vi "Global Var.vi"() -> ()   [LabVIEW 2014]
panel:
  in  "Auto_Cans Delay":bool
  in  "Wips_Auto":bool
  in  "Auto_Cans":bool
  in  "Auto_3_tote":bool
  in  "Auto_Select":bool
  in  "Store_High":bool
  in  "Can_Door":bool
  in  "Master_Auto_Stop":bool
  in  "Yoyo_Pos_Light":dbl
  in  "Light_Show":bool
  in  "Auto 15":bool
  in  "Auto 14":bool
  in  "Auto 13":bool
  in  "Auto 12":bool
  in  "Auto 11":bool
  in  "Auto 10":bool
  in  "Auto 9":bool
  in  "Auto 8":bool
  in  "Auto 7":bool
  in  "Auto 6":bool
  in  "Auto 5":bool
  in  "Auto 4":bool
  in  "Auto 3":bool
  in  "Auto 2":bool
  in  "Auto":bool
  in  "Encoder_Dist":dbl
  in  "Auto_Tote_Picked_Up":bool
  in  "Auto_Infeed_Ben":bool
  in  "Auto_Master_Stop_Value":bool
  in  "Auto_Drive_No_PID_Power":dbl
  in  "Auto_Turn_No_PID_Power":dbl
  in  "Auto_Drive_No_PID_Enable":bool
  in  "Auto_Drive_Straight_Power":dbl
  in  "Auto_Drive_Straight_Enable":bool
  in  "Auto_State":dbl
  in  "Floor_Tote_Detected":bool
  in  "Step_1":bool
  in  "Can_Tip_Flip":bool
  in  "Can_Tip_Arm":bool
  in  "Infeed_Open":bool
  in  "Step_3":bool
  in  "Carry":bool
  in  "Eject_Manual":dbl
  in  "Score_Step":bool
  in  "Score_Tote":dbl
  in  "Reset_Encoder":bool
  in  "Ele_Pos_Yoyo":dbl
  in  "Right_Dist":dbl
  in  "Left_Dist":dbl
  in  "Arm_Pos":bool
  in  "Step_Pos":bool
  in  "Eject_Out":dbl
  in  "Eject_In":dbl
  in  "Reset_Yaw":bool
  in  "Yaw":dbl
  in  "Store_Pos":bool
  in  "Exit_Pos":bool
  in  "Infeed":dbl
  in  "Elevator":dbl
  in  "Station_Pickup":bool
  in  "Floor_Pickup":bool
  in  "Turnin_Main":dbl
  in  "Turning_Limit":dbl
  in  "Speed_Main":dbl
  in  "Speed_Limit":dbl
  # "Auto"
  # "Automation"
  # "Drive Motors"
  # "Sensors"
  # "Positions"
  # "Imp"
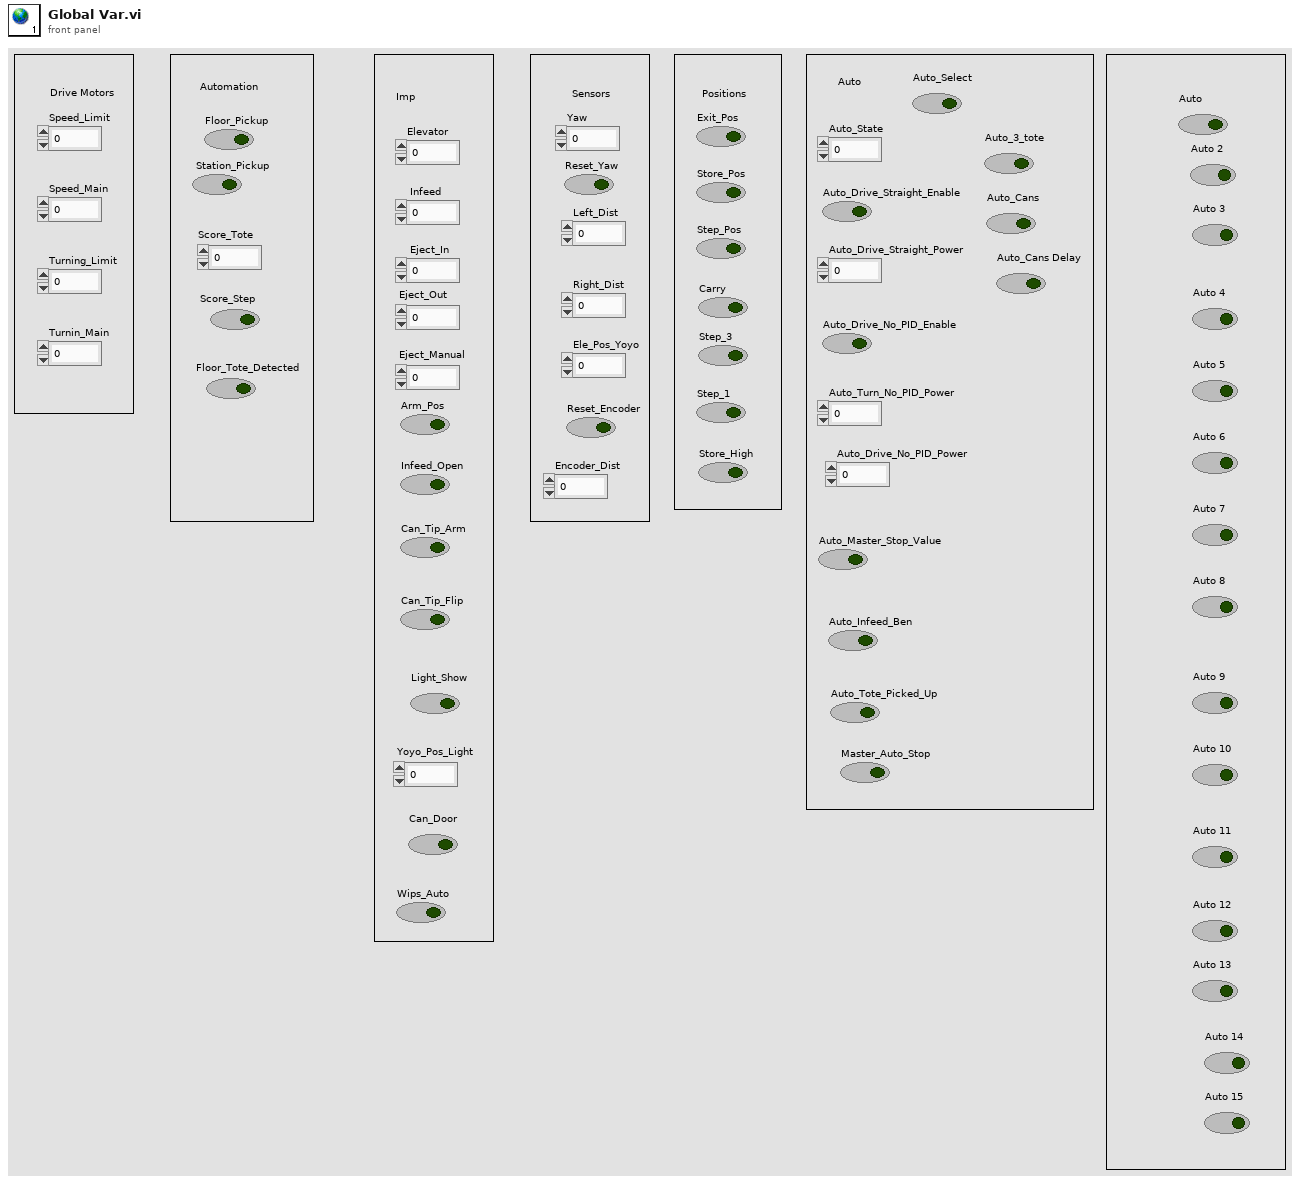
[diagram p1: front panel]
diagram:
